vi "ColorDetection.vi"() -> ()   [LabVIEW 2018]
uses:
  <vilib>/vision/NI_Vision_Development_Module.lvlib
panel:
  out "Blanco":bool
  out "Verde":bool
  out "Azul":bool
  out "Rojo":bool
  out "Color Spectrum":dbl[](array[numeric]) format="%.2f"
  in  "Color Sensitivity":u32(ring) items=["Low", "Medium", "High"]
  in  "Stop (F)":bool
  out "Image Out":T1(plugin-control)
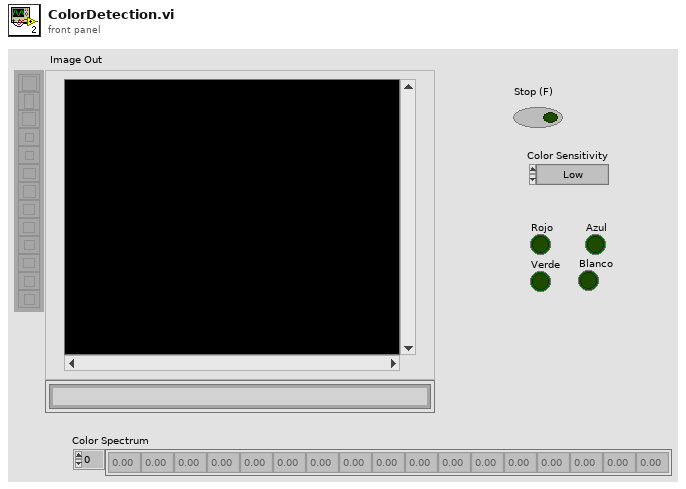
[diagram p1: front panel]
types:
  T1 = typedef "IMAQ Image.ctl" = refnum<image>
  T2 = typedef "IMAQ Rectangle" = cluster{"Left":i32, "Top":i32, "Right":i32, "Bottom":i32, "Rotation":dbl}
  T3 = typedef "ROI Descriptor" = cluster{"Global Rectangle":i32[], "Contours":cluster{"ID":enum32{"External", "Internal"}, "Type":u32, "Coordinates":i32[]}[]}
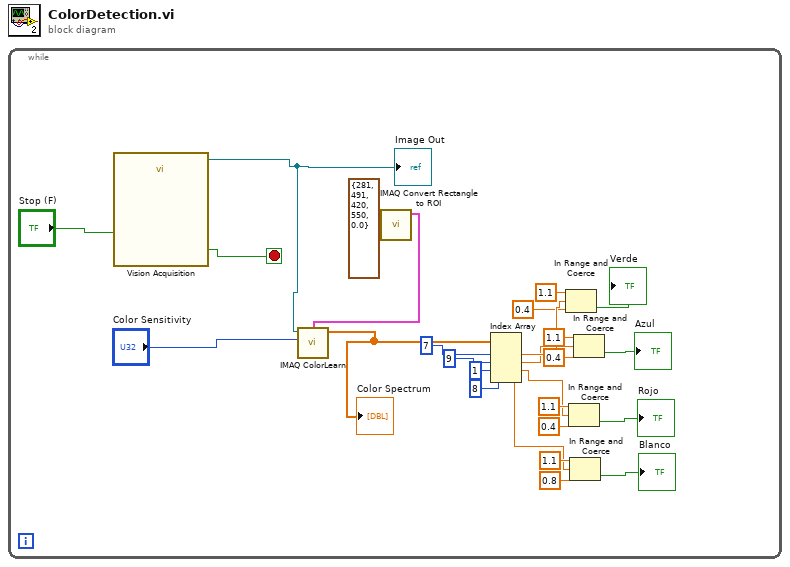
[diagram p0: block diagram]
diagram:
  n1 = while {
    stop <- w26 stop-if-true
    n2 = call "Vision Acquisition"("Stop (F)"="Stop (F)") -> ("Image Out"=w23:T1, "Stopped"=w26:bool)  [unwired: 24 in, 1 out]
    "Image Out" <- w23
    n3 = call "IMAQ Convert Rectangle to ROI"("Rectangle"=T2 {"Left"=281, "Top"=491, "Right"=420, "Bottom"=550, "Rotation"=0.0}) -> ("ROI Descriptor"=w24:T3)  [unwired: 8 in, 1 out]
    n4 = call "IMAQ ColorLearn"("ROI Descriptor"=w24, "Image"=w23, "Color Sensitivity"="Color Sensitivity") -> ("Color Spectrum"=w22:dbl[])  [unwired: 5 in, 1 out]
    "Color Spectrum" <- w22
    n5 = Index Array(array=w22, index #1=7 ("index"), index #2=9 ("index"), index #3=1 ("index"), index #4=8 ("index")) -> (element #1=w17:dbl, element #2=w16:dbl, element #3=w10:dbl, element #4=w1:dbl)
    n6 = In Range and Coerce(upper limit=1.1, x=w17, lower limit=0.4) -> (In Range?=→"Verde":bool)  [unwired: 1 out]
    n7 = In Range and Coerce(upper limit=1.1, x=w10, lower limit=0.4) -> (In Range?=→"Rojo":bool)  [unwired: 1 out]
    n8 = In Range and Coerce(upper limit=1.1, x=w1, lower limit=0.8) -> (In Range?=→"Blanco":bool)  [unwired: 1 out]
    n9 = In Range and Coerce(upper limit=1.1, x=w16, lower limit=0.4) -> (In Range?=→"Azul":bool)  [unwired: 1 out]
  }
